vi "decimal to binary.vi"() -> ()   [LabVIEW 2020]
panel:
  out "Waveform Graph":i16[](graph)
  out "reversed array":i16[](array[numeric])
  in  "Numeric":u8
  out "0, 1":u8[](array[numeric])
  out "Boolean array":bool[](array[boolean])
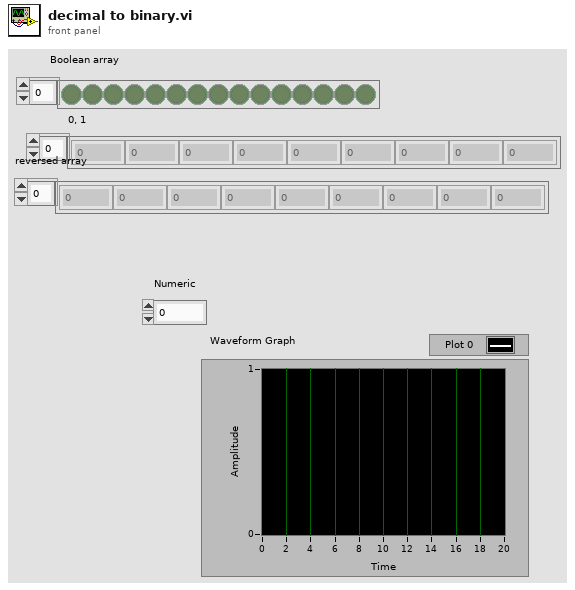
[diagram p1: front panel]
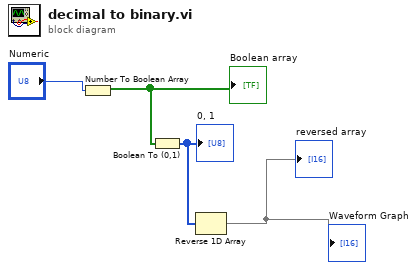
[diagram p0: block diagram]
diagram:
  n1 = Number To Boolean Array(number="Numeric") -> (Boolean array=w4:bool[])
  "Boolean array" <- w4
  n2 = Boolean To (0,1)(Boolean=w4) -> (0, 1=w2:i16[])
  "0, 1" <- w2
  n3 = Reverse 1D Array(array=w2) -> (reversed array=→"reversed array" →"Waveform Graph":i16[])
